vi "Write Measurement Values_Restore to defaults.vi"(0 "Selected Part Name":string="1891", 1 "Ticked Measurement\nIndex":u32[](array[numeric]), 5 "M and N array":T1(array[cluster])=[{"M1"=1, "M2"=2, "N1"=3, "N2"=4}, {"M1"=5, "M2"=6, "N1"=7, "N2"=8}, {"M1"=9, "M2"=10, "N1"=11, "N2"=12}], 7 "Input File Paths Cluster":T3={"JSON Default filepath in"=path "F:/User Interface Testbench/Configuration file/Zengage System JSON UI.json", "JSON RackController\n(Override) filepath in"=path "F:/User Interface Testbench/Configuration file/Rack Controller Override JSON UI.json", "JSON AlgoParameters\n(Override) filepath in"=path "F:/User Interface Testbench/Configuration file/Algorithm Override JSON.json"}, 9 "Measurements Cluster":T2={"Measurement Values"=[["L", "AET", "16", "2", "10", "2", "10", "1", "0"], ["W", "AET", "2.5", "-10", "100", "-10", "100", "1", "0"], ["I1", "Length", "9.5", "-10", "100", "-10", "100", "1", "0"], ["U", "Coord", "2.3", "2", "20", "-10", "100", "1", "0"]], "Enabled Disable Array"=[]}, 11 "error in":errorcluster) -> (4 "RC JSON variant":variant, 6 "Algo JSON variant":variant, 15 "error out":errorcluster)   [LabVIEW 2015]
uses:
  ZenGage v3.0 UI.lvclass
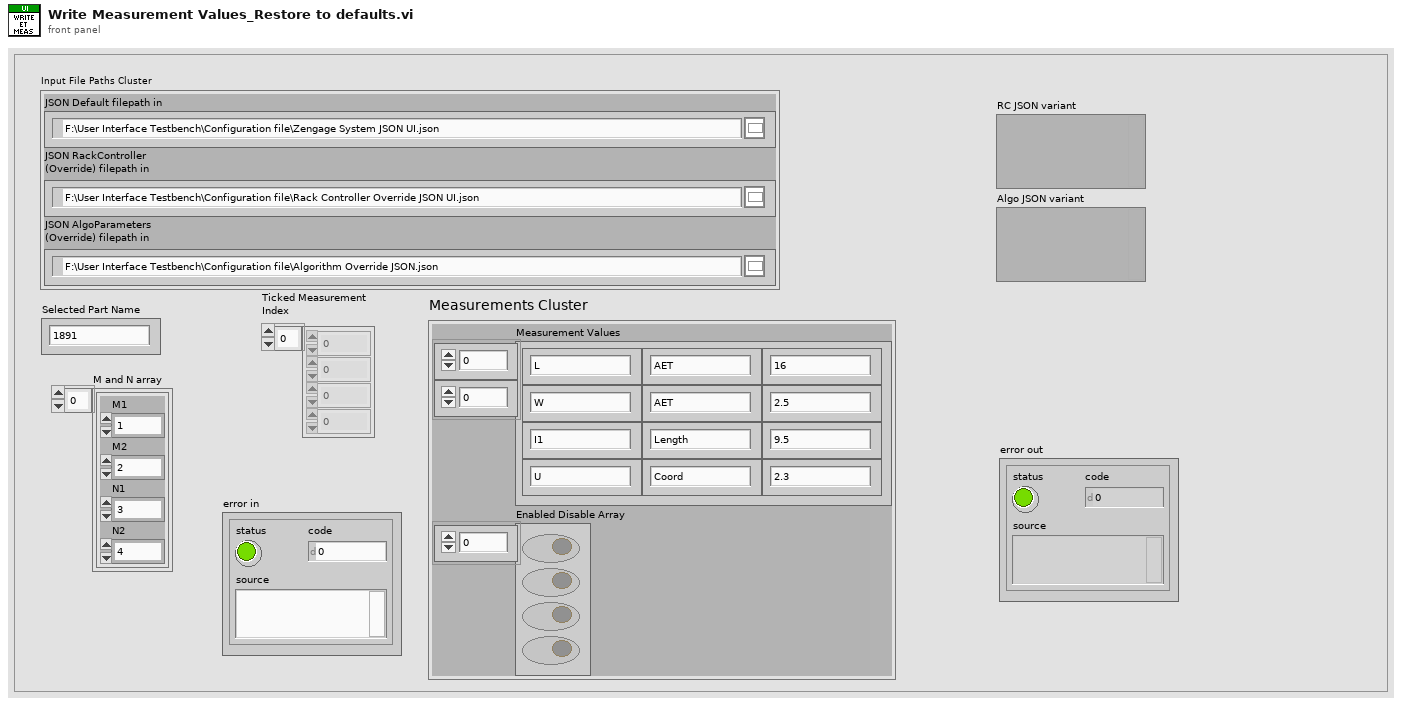
[diagram p1: front panel]
types:
  T1 = cluster{"M1":u64, "M2":u64, "N1":u64, "N2":u64}[]
  T2 = cluster{"Measurement Values":string[][], "Enabled Disable Array":bool[]}
  T3 = cluster{"JSON Default filepath in":path, "JSON RackController\n(Override) filepath in":path, "JSON AlgoParameters\n(Override) filepath in":path}
  T4 = cluster{"Tolerance Limits":dbl[][], "Measurement Enable":bool[], "Bias Correction":dbl[], "Linearity Correction":dbl[], "Measurement names":string[]}
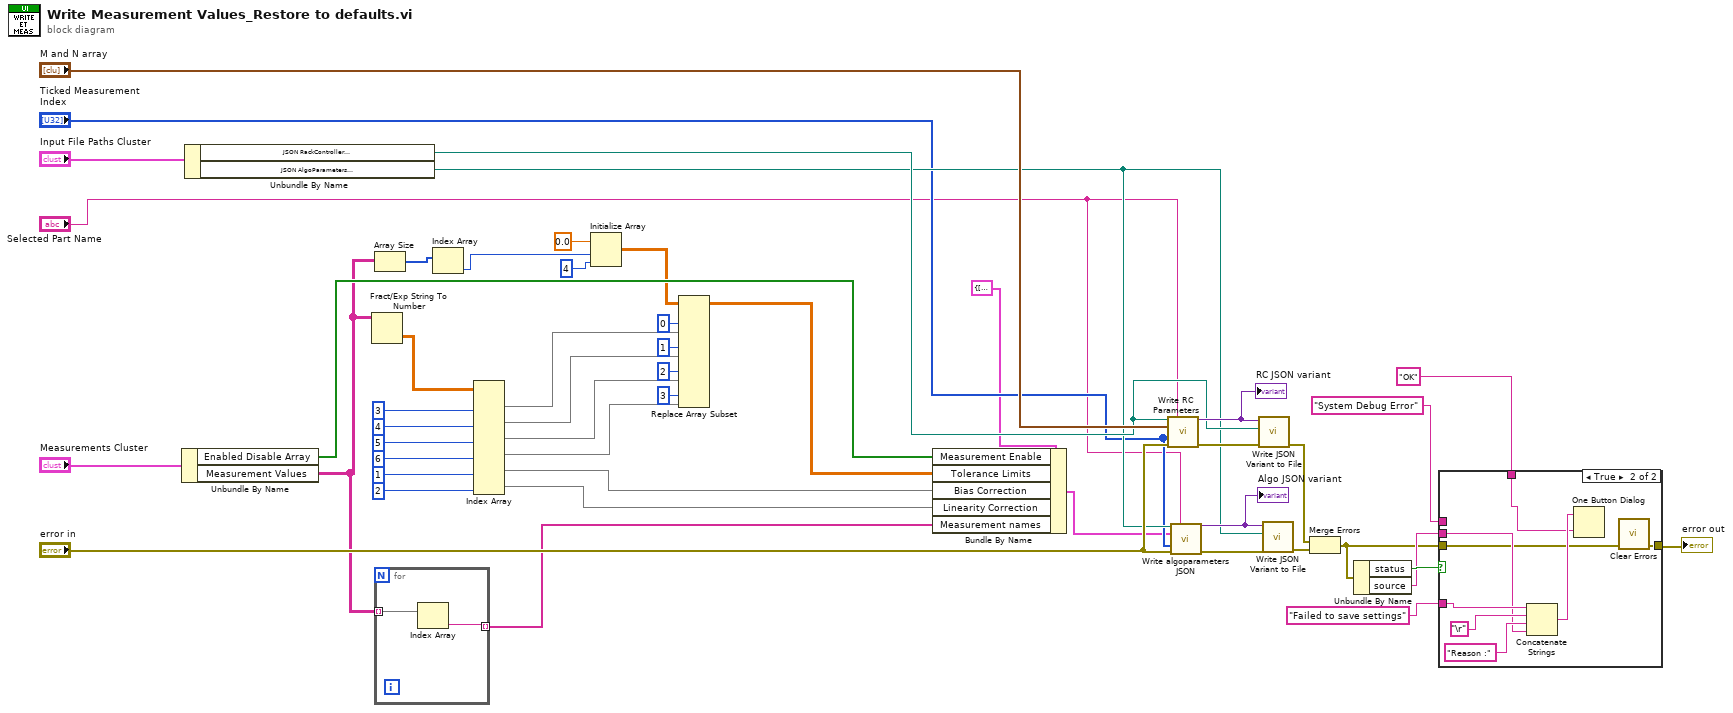
[diagram p0: block diagram]
diagram:
  n1 = Unbundle By Name("Measurements Cluster") -> ("Enabled Disable Array"=w46:bool[], "Measurement Values"=w2:string[][])
  n2 = Unbundle By Name("Input File Paths Cluster") -> ("JSON RackController\n(Override) filepath in"=w32:path, "JSON AlgoParameters\n(Override) filepath in"=w31:path)
  n3 = Fract/Exp String To Number(string=w2) -> (number=w43:dbl[][])  [unwired: 3 in, 1 out]
  n4 = Array Size(array=w2) -> (size(s)=w19:i32[])
  n5 = for {
    tunnel: w2 -> [w51] mode=indexing
    tunnel: [w50] -> w1 mode=indexing
    n6 = Index Array(array=w51) -> (element=w50:string)  [unwired: 1 in]
  }
  n7 = Index Array(array=w19) -> (element=w18:i32)  [unwired: 1 in]
  n8 = Index Array(array=w43, index (col) #1=3 ("index (row)"), index (col) #2=4 ("index (row)"), index (col) #3=5 ("index (row)"), index (col) #4=6 ("index (row)"), index (col) #5=1 ("index (row)"), index (col) #6=2 ("index (row)")) -> (element #1=w42:dbl[], element #2=w41:dbl[], element #3=w40:dbl[], element #4=w39:dbl[], element #5=w28:dbl[], element #6=w27:dbl[])  [unwired: 6 in]
  n9 = Initialize Array(0.0, w18, 4 ("dimension size")) -> (w44:dbl[][])
  n10 = Replace Array Subset(array=w44, new element #1=w42, index (col) #1=0 ("disabled index (col)"), new element #2=w41, index (col) #2=1 ("index (col)"), new element #3=w40, index (col) #3=2 ("index (col)"), new element #4=w39, index (col) #4=3 ("index (col)")) -> (w24:dbl[][])  [unwired: 4 in]
  n11 = Bundle By Name(cluster=T4 {"Tolerance Limits"=[[3.9, 4.3, 3.9, 4.3], [15.2, 15.8, 15.2, 15.8], [15.2, 15.8, 15.2, 15.8], [15.2, 15.8, 15.2, 15.8], [15.2, 15.8, 15.2, 15.8], [15.2, 15.8, 15.2, 15.8], [15.2, 15.8, 15.2, 15.8]], "Measurement Enable"=[TRUE, TRUE, TRUE, TRUE, TRUE, TRUE, TRUE], "Bias Correction"=[-0.144, -0.779, -0.779, -0.779, -0.779, -0.779, -0.779], "Linearity Correction"=[1.0, 1.047, 1.047, 1.047, 1.047, 1.047, 1.047], "Measurement names"=[]} ("Input data cluster"), "Measurement Enable"=w46, "Tolerance Limits"=w24, "Bias Correction"=w28, "Linearity Correction"=w27, "Measurement names"=w1) -> (w3:T4)
  n12 = call "Write RC Parameters.vi"("JSON FilePath"=w32, "Part Name"="Selected Part Name", "M and N array"="M and N array", "Ticked measurements"="Ticked Measurement\nIndex", "error in (no error)"="error in") -> ("JSON Variant"=w33:variant, "error out"=w36:errorcluster)  [unwired: 9 in]
  "RC JSON variant" <- w33
  n13 = call "Write algoparameters JSON.vi"("JSON FilePath"=w31, "Part Name"="Selected Part Name", "Input data cluster"=w3, "Ticked measurements"="Ticked Measurement\nIndex", "error in (no error)"="error in") -> ("JSON Variant"=w34:variant, "error out"=w35:errorcluster)  [unwired: 9 in]
  "Algo JSON variant" <- w34
  n14 = call <vilib>:"Write JSON Variant to File.vi"("Error In"=w36, "file (use dialog)"=w32, "JSON Varaint"=w33) -> ("error out"=w29:errorcluster)  [unwired: 8 in]
  n15 = call <vilib>:"Write JSON Variant to File.vi"("Error In"=w35, "file (use dialog)"=w31, "JSON Varaint"=w34) -> ("error out"=w30:errorcluster)  [unwired: 8 in]
  n16 = Merge Errors(w29, w30) -> (w8:errorcluster)
  n17 = Unbundle By Name(w8) -> ("status"=w10:bool, "source"=w9:string)
  n18 = case shown="True" w10 {
    tunnel: "Failed to save settings" ("Message in") -> [_ w60]
    tunnel: w9 -> [_ w57]
    tunnel: w8 -> [w52 w53]
    tunnel: [w52 w56] -> w5
    tunnel: "System Debug Error" ("Dialogbox header") -> [_ _]
    tunnel: "OK" ("Button Name") -> [_ w54]
    frame False {
    }
    frame True {
      n19 = Concatenate Strings(w60, "\r", "Reason :" ("string"), w57) -> (w55:string)
      n20 = One Button Dialog(message=w55, button name ("OK")=w54) -> ()  [unwired: 1 out]
      n21 = call <vilib>:"Clear Errors.vi"("error in (no error)"=w53) -> ("error out"=w56:errorcluster)  [unwired: 5 in, 1 out]
    }
  }
  "error out" <- w5
